vi "Array_Average_Calculator.vi"() -> ()   [LabVIEW 2026]
panel:
  out "Average":dbl
  out "Number of Elements":i32
  out "Sum":dbl
  in  "Input Array":dbl[](array[numeric])
  # "Array Average Calculator"
  # "Calculates the Sum, number of elements,\nand average of a numeric input array."
  # "Results"
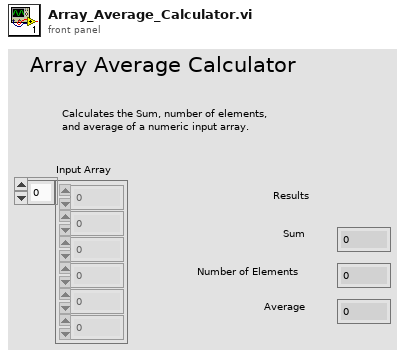
[diagram p1: front panel]
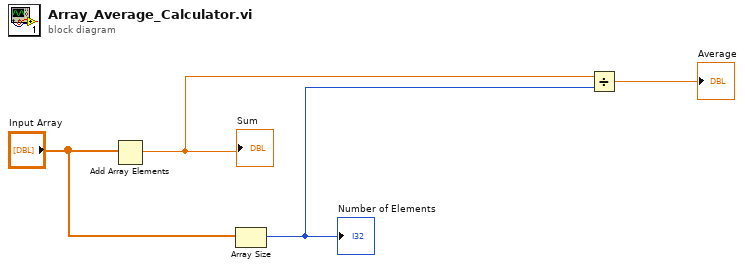
[diagram p0: block diagram]
diagram:
  n1 = Add Array Elements(numeric array="Input Array") -> (sum=w2:dbl)
  "Sum" <- w2
  n2 = Array Size(array="Input Array") -> (size(s)=w3:i32)
  "Number of Elements" <- w3
  n3 = Divide(x=w2, y=w3) -> (x/y=→"Average":dbl)
